vi "s.vi"() -> ()   [LabVIEW 2019]
panel:
  out "Target Position":dbl
  out "backRight":dbl
  out "backLeft":dbl
  out "frontRight":dbl
  out "frontLeft":dbl
  in  "gyroscope position":dbl
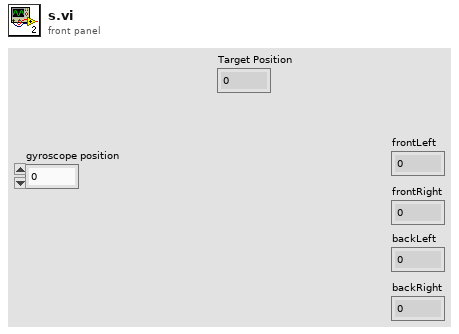
[diagram p1: front panel]
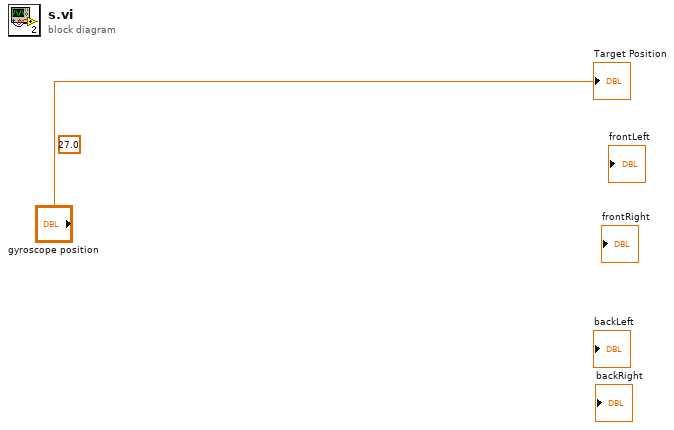
[diagram p0: block diagram]
diagram:
  (unwired) 27.0
  "Target Position" <- "gyroscope position"
